vi "Timer.vi"(8 "error in (no error)":errorcluster, 9 "Time Target(s)":dbl=10.0 format="%#_13g", 10 "Reset":bool, 11 "Pause":bool) -> (0 "error out":errorcluster, 1 "Elapsed TIme":dbl, 2 "Elapsed?":bool)   [LabVIEW 2013]
doc: "This subVI has following funcnality\n1.Pause- When it is pressed it stops the running elapsed time to the current value.\n2.Reset- Change the elapsed time value to zero.\n3.Elapsed; On- Time is elapsed\n Off- Time has not elapsed.\n4.Elapsed Time- Count the elapsed time"
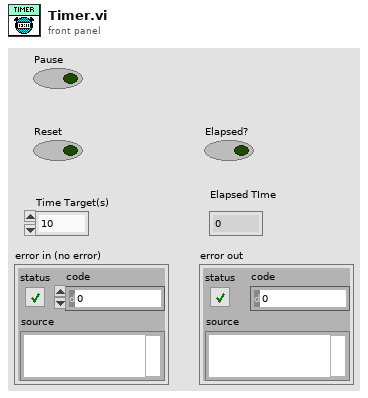
[diagram p1: front panel]
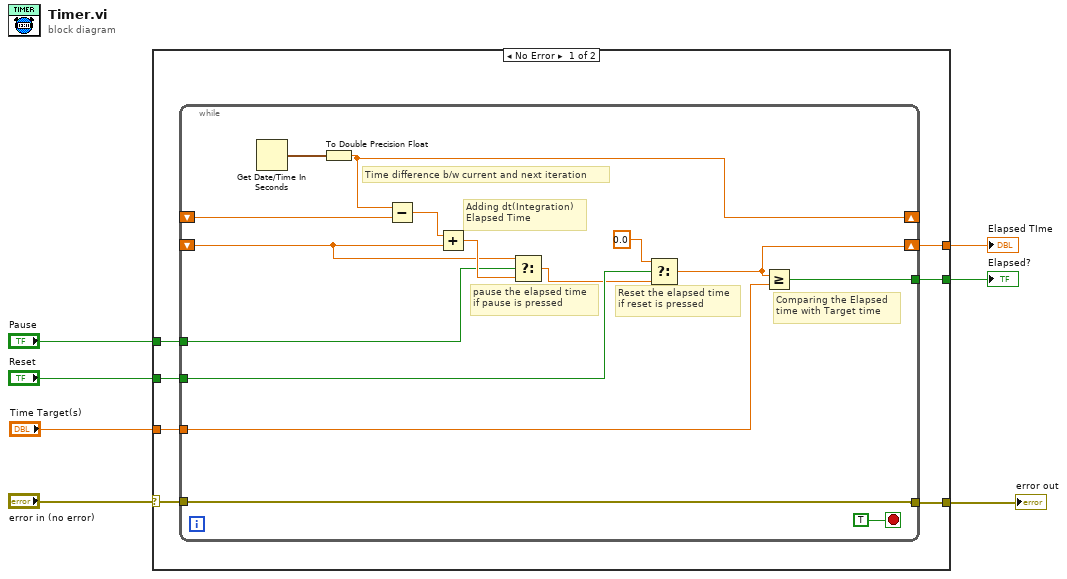
[diagram p0: block diagram]
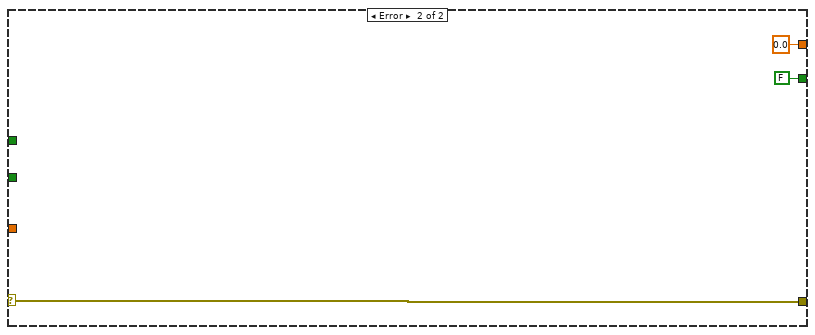
[diagram p2: hidden frame]
diagram:
  n1 = case shown="No Error" "error in (no error)" {
    selector: "error in (no error)" -> [w10 w32]
    tunnel: [w14 0.0 ("t")] -> w2
    tunnel: [w13 FALSE] -> w3
    tunnel: "Reset" -> [w12 _]
    tunnel: "Pause" -> [w11 _]
    tunnel: [w9 w32] -> w7
    tunnel: "Time Target(s)" -> [w8 _]
    frame No Error {
      n2 = while {
        shift-right: [w27] -> _
        shift-left: _ -> [w28]
        shift-right: [w24] -> w14
        shift-left: _ -> [w21]
        tunnel: [w17] -> w13
        tunnel: w12 -> [w25]
        tunnel: w11 -> [w19]
        tunnel: w10 -> [w18]
        tunnel: [w18] -> w9
        tunnel: w8 -> [w15]
        stop <- TRUE stop-if-true
        # "Comparing the Elapsed\ntime with Target time"
        # "Reset the elapsed time \nif reset is pressed"
        # "pause the elapsed time \nif pause is pressed"
        # "Adding dt(Integration)\nElapsed Time"
        # "Time difference b/w current and next iteration"
        n3 = Get Date/Time In Seconds() -> (seconds since 1Jan1904=w29:timestamp)
        n4 = To Double Precision Float(number=w29) -> (double precision float=w27:dbl)
        n5 = Subtract(x=w27, y=w28) -> (x-y=w26:dbl)
        n6 = Add(x=w26, y=w21) -> (x+y=w22:dbl)
        n7 = Select(t=w21, s=w19, f=w22) -> (s? t:f=w20:dbl)
        n8 = Select(t=0.0, s=w25, f=w20) -> (s? t:f=w24:dbl)
        n9 = Greater Or Equal?(x=w24, y=w15) -> (x >= y?=w17:bool)
      }
    }
    frame Error {
    }
  }
  "error out" <- w7
  "Elapsed?" <- w3
  "Elapsed TIme" <- w2
